vi "test_libssh2_session_init.vi"() -> ()   [LabVIEW 2013, in "libssh2_tests.lvlib"]
uses:
  libssh2/libssh2_init_default.vi
  libssh2_tests.lvlib
  libssh2/libssh2.lvlib
  <vilib>/addons/_JKI Toolkits/Caraya/classes/Test/Test.lvclass
  <vilib>/addons/_JKI Toolkits/Caraya/classes/Assert/Assert.lvclass
panel:
  out "error out":errorcluster
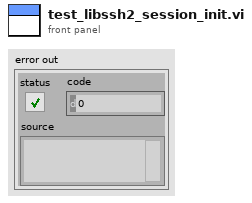
[diagram p1: front panel]
types:
  T1 = typedef "libssh2.lvlib/Session Refnum.ctl" = refnum<k1>
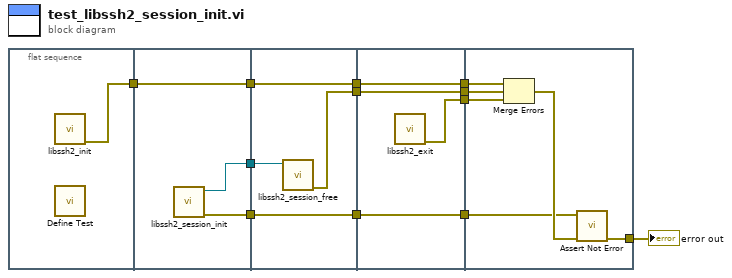
[diagram p0: block diagram]
diagram:
  n1 = flat-sequence {
    tunnel: [w13] -> w7
    tunnel: w7 -> [w16]
    tunnel: [w16] -> w3
    tunnel: [w15] -> w2
    tunnel: [w14] -> w1
    tunnel: w3 -> [w20]
    tunnel: [w20] -> w6
    tunnel: [w19] -> w5
    tunnel: [w18] -> w4
    tunnel: w2 -> [w18]
    tunnel: w1 -> [w17]
    tunnel: w6 -> [w24]
    tunnel: [w24] -> w12
    tunnel: [w23] -> w11
    tunnel: [w22] -> w10
    tunnel: w5 -> [w22]
    tunnel: [w21] -> w8
    tunnel: w4 -> [w21]
    tunnel: w12 -> [w30]
    tunnel: w11 -> [w29]
    tunnel: [w27] -> w9
    tunnel: w10 -> [w26]
    tunnel: w8 -> [w25]
    frame #0 {
      n2 = call-poly "libssh2_init.vi"() -> ("error out"=w13:errorcluster)  [unwired: 11 in]
      n3 = call <vilib>:"Define Test.vi"() -> ()  [unwired: 10 in, 2 out]
    }
    frame #1 {
      n4 = call "libssh2_session_init.vi"() -> ("error out"=w15:errorcluster, "session"=w14:T1)  [unwired: 10 in]
    }
    frame #2 {
      n5 = call "libssh2_session_free.vi"("session"=w17) -> ("error out"=w19:errorcluster)  [unwired: 10 in]
    }
    frame #3 {
      n6 = call "libssh2_exit.vi"() -> ("error out"=w23:errorcluster)  [unwired: 11 in]
    }
    frame #4 {
      n7 = Merge Errors(w30, w26, w29) -> (w28:errorcluster)
      n8 = call <vilib>:"Assert Not Error.vi"("error in (no error)"=w28, "Not Error?"=w25) -> ("error out"=w27:errorcluster)  [unwired: 8 in, 1 out]
    }
  }
  "error out" <- w9
